vi "find_first_and_last_pixel_per_row.vi"(8 "safety margin":i32, 11 "u8_ar_mask":u8[][](array[numeric])) -> (3 "i32_ar_first_and_last_pixel":i32[][](array[numeric]))   [LabVIEW 2011]
doc: "Returns a 2D array containing the first and last pixel per row that contains image information, i.e. that is not masked. Uses the u8_ar_mask from the global variables, so ensure that you write the correct mask information before calling this vi."
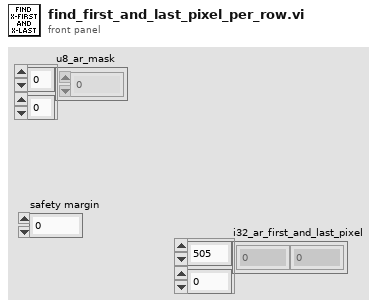
[diagram p1: front panel]
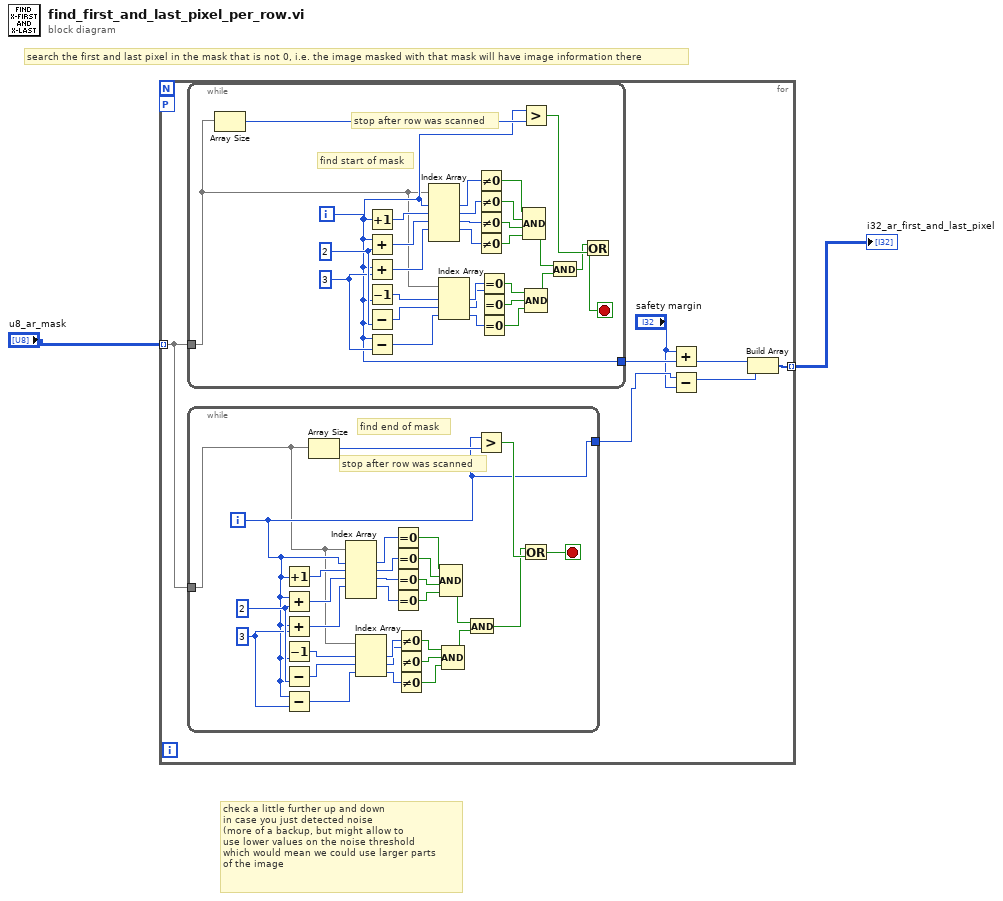
[diagram p0: block diagram]
diagram:
  # "check a little further up and down\nin case you just detected noise\n(more of a backup, but might allow to \nuse lower values on the noise threshold \nwhich would mean we could use larger parts \nof the image"
  # "search the first and last pixel in the mask that is not 0, i.e. the image masked with that mask will have image information there"
  n1 = for {
    tunnel: "u8_ar_mask" -> [w8] mode=indexing
    tunnel: [w9] -> w2 mode=indexing
    workers-P: _ -> [_]
    n2 = while {
      tunnel: w8 -> [w49]
      tunnel: [w50] -> w7
      i -> [w50]
      stop <- w67 stop-if-true
      w51 = 3 ("y")
      w63 = 2 ("y")
      # "stop after row was scanned"
      # "find start of mask"
      n3 = Array Size(array=w49) -> (size(s)=w69:i32)
      n4 = Increment(x=w50) -> (x+1=w59:i32)
      n5 = Add(x=w50, y=w63) -> (x+y=w58:i32)
      n6 = Add(x=w50, y=w51) -> (x+y=w56:i32)
      n7 = Decrement(x=w50) -> (x-1=w57:i32)
      n8 = Subtract(x=w50, y=w63) -> (x-y=w60:i32)
      n9 = Subtract(x=w50, y=w51) -> (x-y=w52:i32)
      n10 = Index Array(array=w49, index #1=w50, index #2=w59, index #3=w58, index #4=w56) -> (element #1=w55:u8, element #2=w54:u8, element #3=w65:u8, element #4=w62:u8)  [unwired: 1 in, 1 out]
      n11 = Index Array(array=w49, index #1=w57, index #2=w60, index #3=w52) -> (element #1=w48:u8, element #2=w46:u8, element #3=w47:u8)
      n12 = Not Equal To 0?(x=w55) -> (x != 0?=w66:bool)
      n13 = Not Equal To 0?(x=w54) -> (x != 0?=w53:bool)
      n14 = Not Equal To 0?(x=w65) -> (x != 0?=w64:bool)
      n15 = Not Equal To 0?(x=w62) -> (x != 0?=w61:bool)
      n16 = Equal To 0?(x=w48) -> (x = 0?=w43:bool)
      n17 = Equal To 0?(x=w46) -> (x = 0?=w44:bool)
      n18 = Equal To 0?(x=w47) -> (x = 0?=w45:bool)
      n19 = Greater?(x=w50, y=w69) -> (0:w68:bool)
      n20 = Compound Arithmetic op=AND(w66, w53, w64, w61) -> (w41:bool)
      n21 = Compound Arithmetic op=AND(w43, w44, w45) -> (w42:bool)
      n22 = And(x=w41, y=w42) -> (x .and. y?=w40:bool)
      n23 = Or(x=w40, y=w68) -> (x .or. y?=w67:bool)
    }
    n24 = while {
      tunnel: [w12] -> w4
      tunnel: w8 -> [w11]
      i -> [w12]
      stop <- w37 stop-if-true
      w21 = 3 ("y")
      w33 = 2 ("y")
      # "find end of mask"
      # "stop after row was scanned"
      n25 = Increment(x=w12) -> (x+1=w29:i32)
      n26 = Add(x=w12, y=w33) -> (x+y=w28:i32)
      n27 = Add(x=w12, y=w21) -> (x+y=w26:i32)
      n28 = Decrement(x=w12) -> (x-1=w27:i32)
      n29 = Subtract(x=w12, y=w33) -> (x-y=w30:i32)
      n30 = Subtract(x=w12, y=w21) -> (x-y=w22:i32)
      n31 = Array Size(array=w11) -> (size(s)=w38:i32)
      n32 = Index Array(array=w11, index #1=w12, index #2=w29, index #3=w28, index #4=w26) -> (element #1=w25:u8, element #2=w24:u8, element #3=w35:u8, element #4=w32:u8)  [unwired: 1 in, 1 out]
      n33 = Index Array(array=w11, index #1=w27, index #2=w30, index #3=w22) -> (element #1=w20:u8, element #2=w18:u8, element #3=w19:u8)
      n34 = Equal To 0?(x=w25) -> (x = 0?=w36:bool)
      n35 = Equal To 0?(x=w24) -> (x = 0?=w23:bool)
      n36 = Equal To 0?(x=w35) -> (x = 0?=w34:bool)
      n37 = Equal To 0?(x=w32) -> (x = 0?=w31:bool)
      n38 = Not Equal To 0?(x=w20) -> (x != 0?=w15:bool)
      n39 = Not Equal To 0?(x=w18) -> (x != 0?=w16:bool)
      n40 = Not Equal To 0?(x=w19) -> (x != 0?=w17:bool)
      n41 = Compound Arithmetic op=AND(w36, w23, w34, w31) -> (w13:bool)
      n42 = Compound Arithmetic op=AND(w15, w16, w17) -> (w14:bool)
      n43 = And(x=w13, y=w14) -> (x .and. y?=w10:bool)
      n44 = Greater?(x=w12, y=w38) -> (0:w39:bool)
      n45 = Or(x=w10, y=w39) -> (x .or. y?=w37:bool)
    }
    n46 = Add(x="safety margin", y=w7) -> (x+y=w6:i32)
    n47 = Subtract(x=w4, y="safety margin") -> (x-y=w5:i32)
    n48 = Build Array(w6, w5) -> (w9:i32[])
  }
  "i32_ar_first_and_last_pixel" <- w2
